vi "Write Export Artifacts for SCC.vi"(8 "error in (no error)":errorcluster, 10 "Export Artifacts for SCC":path[](array[path]), 11 "Export in":refnum<class "Export.lvclass">) -> (0 "error out":errorcluster, 3 "Export out":refnum<class "Export.lvclass">)   [LabVIEW 2017, in "CL_G3_VIComponentBuilder.lvlib" / "Export.lvclass"]
uses:
  Export.lvclass
  Export.lvclass/Export.ctl
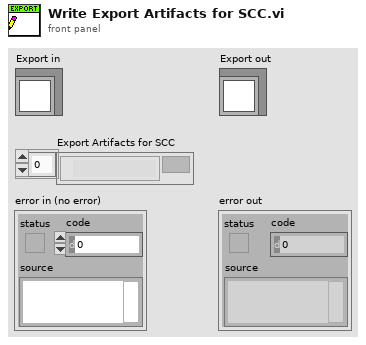
[diagram p1: front panel]
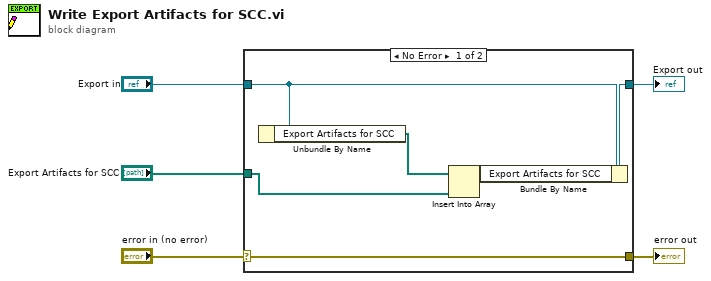
[diagram p0: block diagram]
diagram:
  n1 = case shown="No Error" "error in (no error)" {
    selector: "error in (no error)" -> [w11 w12]
    tunnel: [w11 w12] -> w4
    tunnel: [w10 w13] -> w2
    tunnel: "Export in" -> [w9 w13]
    tunnel: "Export Artifacts for SCC" -> [w8 _]
    frame No Error {
      n2 = Unbundle By Name(w9) -> ("Export Artifacts for SCC"=w6:path[])
      n3 = Insert Into Array(array=w6, new element=w8) -> (w7:path[])  [unwired: 1 in]
      n4 = Bundle By Name(cluster=w9, "Export Artifacts for SCC"=w7) -> (w10:refnum<class "Export.lvclass">)
    }
    frame Error {
    }
  }
  "error out" <- w4
  "Export out" <- w2
